vi "Get Clone ID.vi"(11 "Process in":refnum<class "Process.lvclass">) -> (3 "Process out":refnum<class "Process.lvclass">)   [LabVIEW 2020, in "Process.lvclass"]
uses:
  Process.lvclass
  Process.lvclass/Process.ctl
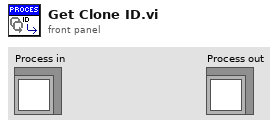
[diagram p1: front panel]
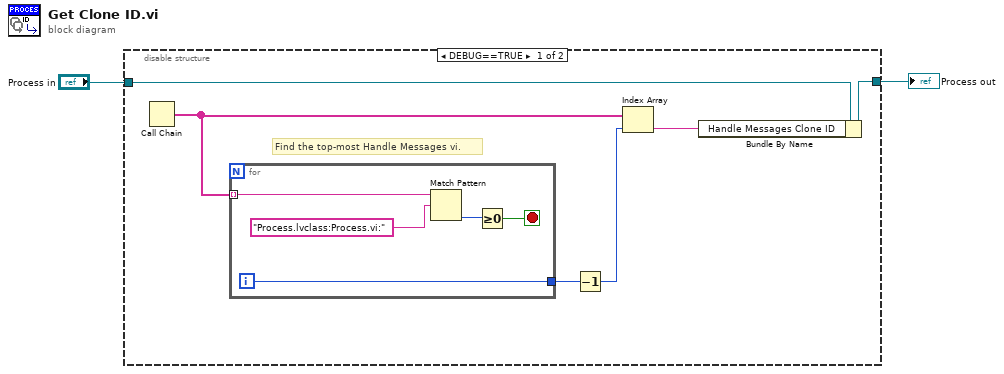
[diagram p0: block diagram]
diagram:
  n1 = disable-structure shown="DEBUG==TRUE" {
    disable-tunnel: [w8 w14] -> w2
    disable-tunnel: "Process in" -> [w7 w14]
    frame condition #0 (active) {
      # "Find the top-most Handle Messages vi."
      n2 = Call Chain() -> (call chain=w5:string[])
      n3 = for {
        tunnel: w5 -> [w13] mode=indexing
        tunnel: [w9] -> w4
        i -> [w9]
        stop <- w10 stop-if-true
        n4 = Match Pattern(string=w13, regular expression="Process.lvclass:Process.vi:") -> (offset past match=w11:i32)  [unwired: 1 in, 3 out]
        n5 = Greater Or Equal To 0?(x=w11) -> (x >= 0?=w10:bool)
      }
      n6 = Decrement(x=w4) -> (x-1=w3:i32)
      n7 = Index Array(array=w5, index=w3) -> (element=w6:string)
      n8 = Bundle By Name(cluster=w7, "Handle Messages Clone ID"=w6) -> (w8:refnum<class "Process.lvclass">)
    }
    frame condition #1 {
    }
  }
  "Process out" <- w2
